vi "Maquina_de_estados_Tarea.vi"() -> ()   [LabVIEW 2024]
panel:
  out "C. Gruesa":dbl
  out "C. Delgada":dbl
  out "Taladro":dbl(slide)
  in  "stop":bool
  out "A3":bool
  out "A2":bool
  out "A1":bool
  out "A0":bool
  out "Delgada":bool
  out "Prendido":bool
  out "Apagado":bool
  in  "Inicio":bool
  out "Gruesa":bool
  in  "SH":bool
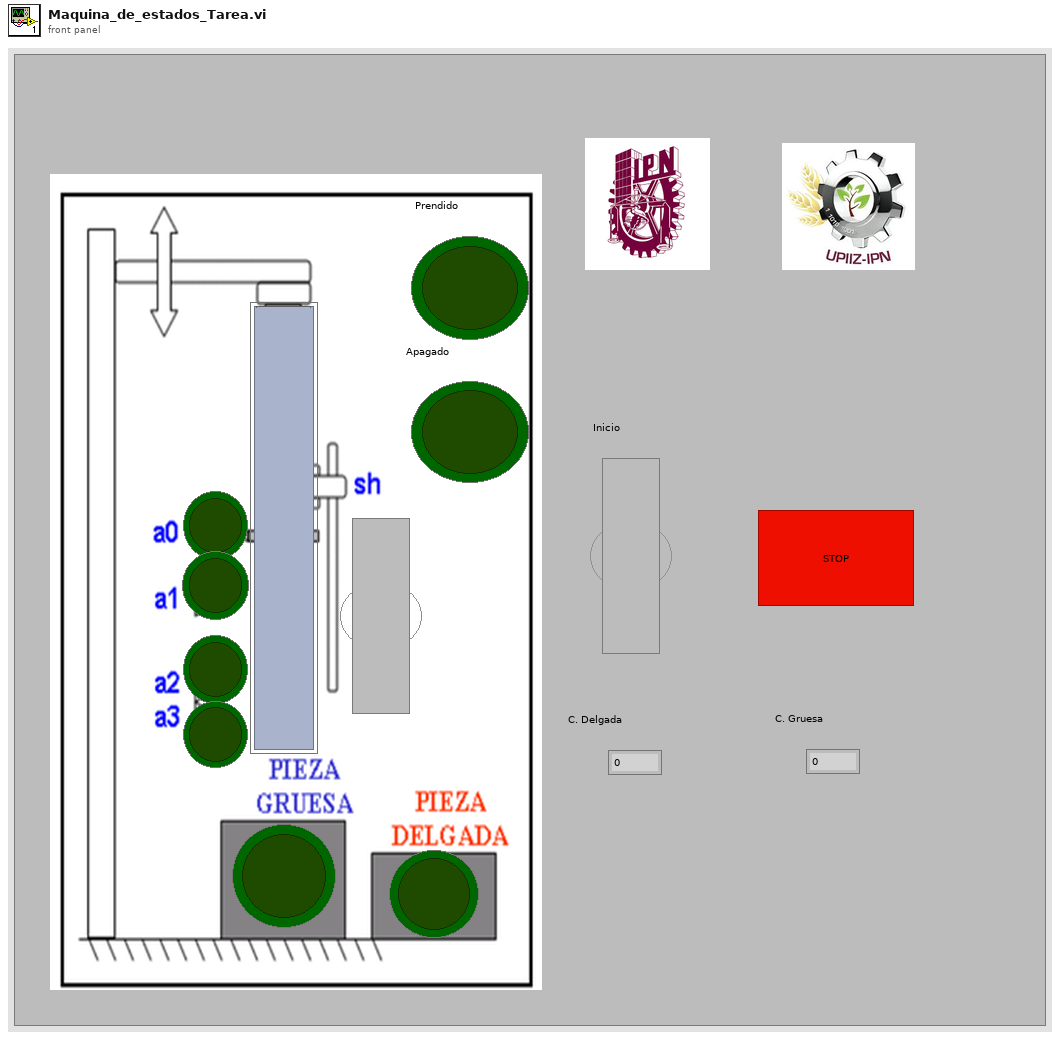
[diagram p1: front panel]
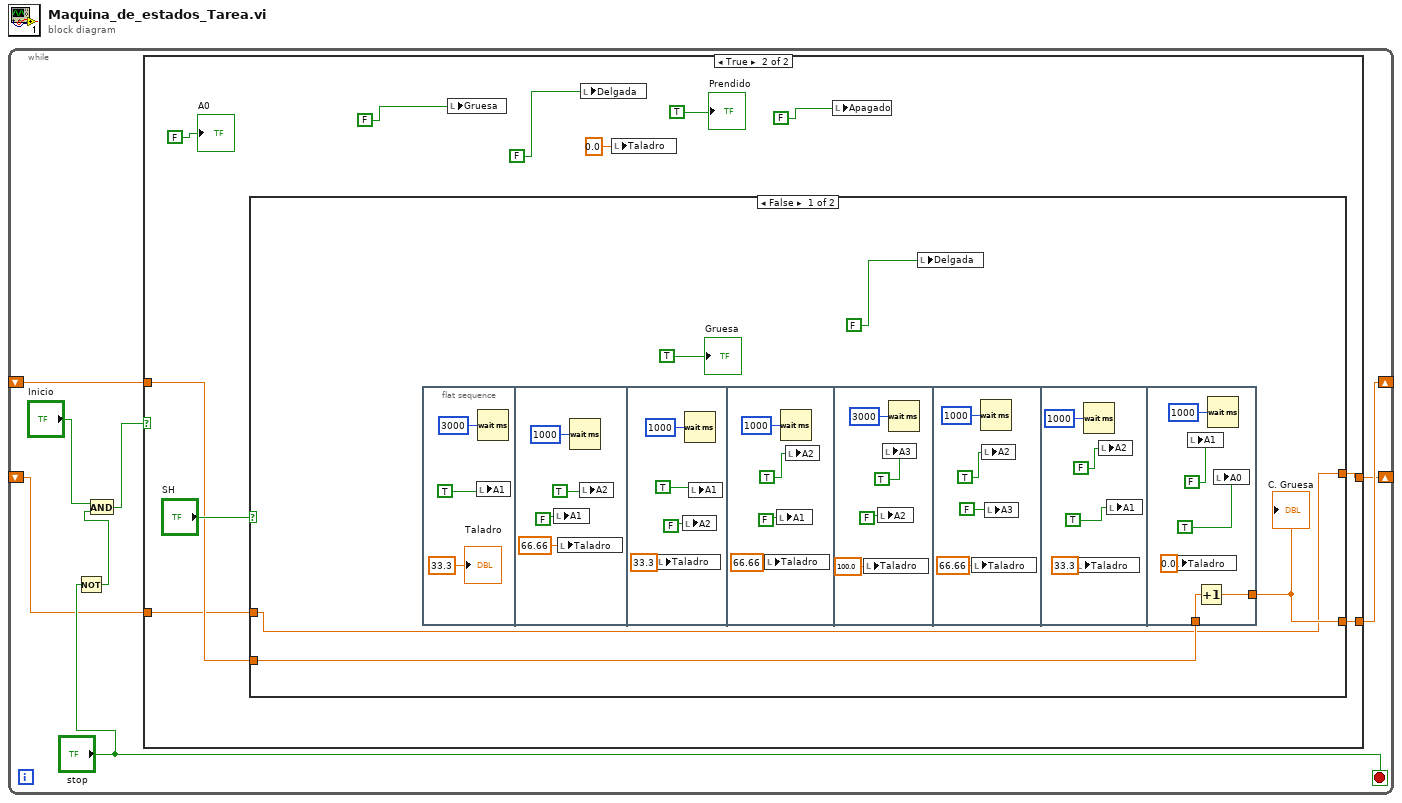
[diagram p0: block diagram]
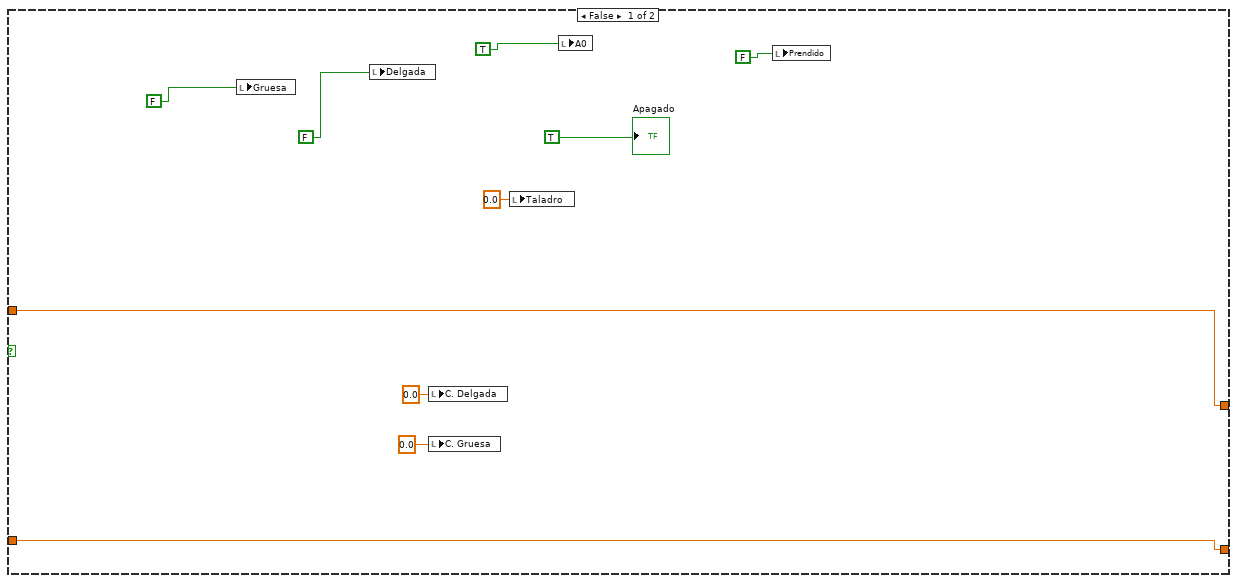
[diagram p2: hidden frame]
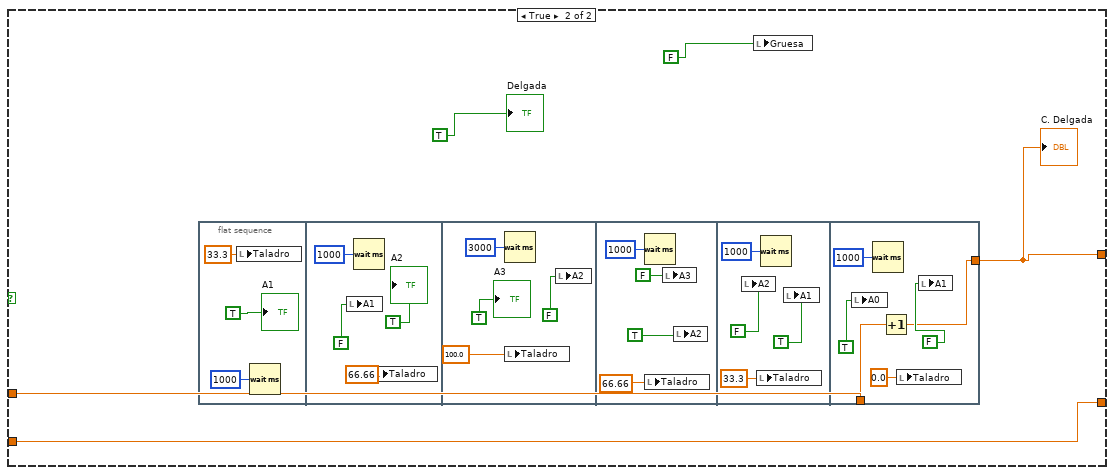
[diagram p3: hidden frame]
diagram:
  n1 = while {
    shift-right: [w3] -> _
    shift-left: _ -> [w4]
    shift-right: [w2] -> _
    shift-left: _ -> [w1]
    stop <- "stop" stop-if-true
    n2 = Not(x="stop") -> (.not. x?=w8:bool)
    n3 = And(x="Inicio", y=w8) -> (x .and. y?=w7:bool)
    n4 = case shown="True" w7 {
      tunnel: w4 -> [w14 w24]
      tunnel: [w13 w23] -> w3
      tunnel: [w14 w22] -> w2
      tunnel: w1 -> [w13 w21]
      frame False {
        n5 = local write "Gruesa"(FALSE) -> ()
        n6 = local write "Delgada"(FALSE) -> ()
        n7 = local write "C. Delgada"(0.0 ("C. Delgada")) -> ()
        n8 = local write "C. Gruesa"(0.0 ("C. Delgada")) -> ()
        n9 = local write "Taladro"(0.0 ("Taladro")) -> ()
        n10 = local write "A0"(TRUE) -> ()
        n11 = local write "Prendido"(FALSE) -> ()
        "Apagado" <- TRUE
      }
      frame True {
        n12 = case shown="False" "SH" {
          tunnel: w24 -> [w32 w68]
          tunnel: [w31 w68] -> w23
          tunnel: [w30 w70] -> w22
          tunnel: w21 -> [w30 w69]
          frame False {
            n13 = flat-sequence {
              tunnel: w32 -> [w63]
              tunnel: [w62] -> w31
              frame #0 {
                n14 = local write "A1"(TRUE) -> ()
                n15 = Wait (ms)(milliseconds to wait=u32 3000) -> ()  [unwired: 1 out]
                "Taladro" <- 33.3 ("Taladro")
              }
              frame #1 {
                n16 = local write "A1"(FALSE) -> ()
                n17 = local write "Taladro"(66.66 ("Taladro")) -> ()
                n18 = Wait (ms)(milliseconds to wait=u32 1000) -> ()  [unwired: 1 out]
                n19 = local write "A2"(TRUE) -> ()
              }
              frame #2 {
                n20 = local write "Taladro"(33.3 ("Taladro")) -> ()
                n21 = local write "A2"(FALSE) -> ()
                n22 = Wait (ms)(milliseconds to wait=u32 1000) -> ()  [unwired: 1 out]
                n23 = local write "A1"(TRUE) -> ()
              }
              frame #3 {
                n24 = local write "Taladro"(66.66 ("Taladro")) -> ()
                n25 = local write "A1"(FALSE) -> ()
                n26 = Wait (ms)(milliseconds to wait=u32 1000) -> ()  [unwired: 1 out]
                n27 = local write "A2"(TRUE) -> ()
              }
              frame #4 {
                n28 = local write "Taladro"(100.0 ("Taladro")) -> ()
                n29 = local write "A2"(FALSE) -> ()
                n30 = local write "A3"(TRUE) -> ()
                n31 = Wait (ms)(milliseconds to wait=u32 3000) -> ()  [unwired: 1 out]
              }
              frame #5 {
                n32 = local write "Taladro"(66.66 ("Taladro")) -> ()
                n33 = Wait (ms)(milliseconds to wait=u32 1000) -> ()  [unwired: 1 out]
                n34 = local write "A2"(TRUE) -> ()
                n35 = local write "A3"(FALSE) -> ()
              }
              frame #6 {
                n36 = local write "Taladro"(33.3 ("Taladro")) -> ()
                n37 = Wait (ms)(milliseconds to wait=u32 1000) -> ()  [unwired: 1 out]
                n38 = local write "A2"(FALSE) -> ()
                n39 = local write "A1"(TRUE) -> ()
              }
              frame #7 {
                n40 = local write "Taladro"(0.0 ("Taladro")) -> ()
                n41 = local write "A1"(FALSE) -> ()
                n42 = Increment(x=w63) -> (x+1=w62:dbl)
                n43 = Wait (ms)(milliseconds to wait=u32 1000) -> ()  [unwired: 1 out]
                n44 = local write "A0"(TRUE) -> ()
              }
            }
            n45 = local write "Delgada"(FALSE) -> ()
            "Gruesa" <- TRUE
            "C. Gruesa" <- w31
          }
          frame True {
            n46 = flat-sequence {
              tunnel: [w93] -> w70
              tunnel: w69 -> [w92]
              frame #0 {
                n47 = local write "Taladro"(33.3 ("Taladro")) -> ()
                n48 = Wait (ms)(milliseconds to wait=u32 1000) -> ()  [unwired: 1 out]
                "A1" <- TRUE
              }
              frame #1 {
                n49 = local write "A1"(FALSE) -> ()
                n50 = Wait (ms)(milliseconds to wait=u32 1000) -> ()  [unwired: 1 out]
                n51 = local write "Taladro"(66.66 ("Taladro")) -> ()
                "A2" <- TRUE
              }
              frame #2 {
                n52 = Wait (ms)(milliseconds to wait=u32 3000) -> ()  [unwired: 1 out]
                n53 = local write "Taladro"(100.0 ("Taladro")) -> ()
                n54 = local write "A2"(FALSE) -> ()
                "A3" <- TRUE
              }
              frame #3 {
                n55 = Wait (ms)(milliseconds to wait=u32 1000) -> ()  [unwired: 1 out]
                n56 = local write "Taladro"(66.66 ("Taladro")) -> ()
                n57 = local write "A3"(FALSE) -> ()
                n58 = local write "A2"(TRUE) -> ()
              }
              frame #4 {
                n59 = local write "A2"(FALSE) -> ()
                n60 = local write "Taladro"(33.3 ("Taladro")) -> ()
                n61 = Wait (ms)(milliseconds to wait=u32 1000) -> ()  [unwired: 1 out]
                n62 = local write "A1"(TRUE) -> ()
              }
              frame #5 {
                n63 = local write "A0"(TRUE) -> ()
                n64 = Wait (ms)(milliseconds to wait=u32 1000) -> ()  [unwired: 1 out]
                n65 = Increment(x=w92) -> (x+1=w93:dbl)
                n66 = local write "Taladro"(0.0 ("Taladro")) -> ()
                n67 = local write "A1"(FALSE) -> ()
              }
            }
            n68 = local write "Gruesa"(FALSE) -> ()
            "Delgada" <- TRUE
            "C. Delgada" <- w70
          }
        }
        n69 = local write "Gruesa"(FALSE) -> ()
        n70 = local write "Delgada"(FALSE) -> ()
        n71 = local write "Taladro"(0.0 ("Taladro")) -> ()
        n72 = local write "Apagado"(FALSE) -> ()
        "A0" <- FALSE
        "Prendido" <- TRUE
      }
    }
  }
